vi "Event Handle Loop_Origin Zero.vi"(8 "error in (no error)":errorcluster, 11 "QTab Class in":refnum<class "QTab Class.lvclass">) -> (0 "error out":errorcluster, 3 "QTab Class out":refnum<class "QTab Class.lvclass">)   [LabVIEW 2020, in "QTab.lvlib" / "QTab Class.lvclass"]
uses:
  QTab Class.lvclass
  <vilib>/Utility/miscctls.llb/LVPointTypeDef.ctl
  QTab Class.lvclass/QTab Class.ctl
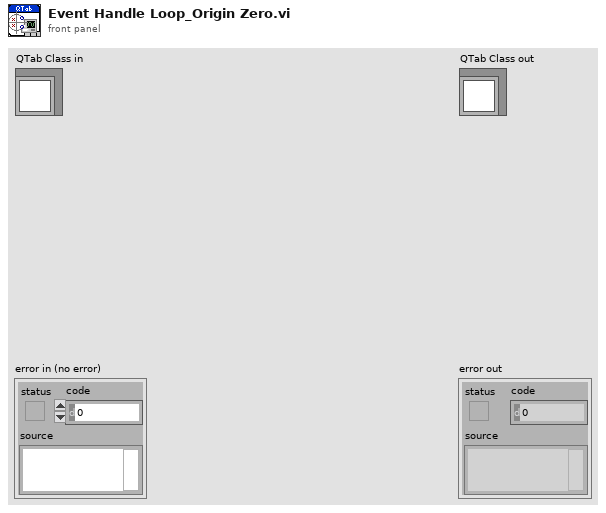
[diagram p1: front panel]
types:
  T1 = typedef "LVPointTypeDef.ctl" = cluster{"Horizontal":i16, "Vertical":i16}
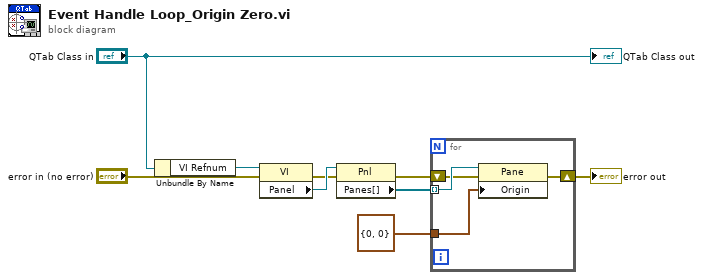
[diagram p0: block diagram]
diagram:
  n1 = Unbundle By Name("QTab Class in") -> ("VI Refnum"=w3:refnum<vi>)
  n2 = property class="VI"(reference=w3, error in="error in (no error)") -> (error out=w7:errorcluster, "Panel"=w9:refnum<vi>)  [unwired: 1 out]
  n3 = property class="Pnl"(reference=w9, error in=w7) -> (error out=w2:errorcluster, "Panes[]"=w8:refnum<vi>[])  [unwired: 1 out]
  n4 = for {
    tunnel: w8 -> [w13] mode=indexing
    shift-right: [w12] -> w1
    shift-left: w2 -> [w11]
    tunnel: T1 {"Horizontal"=0, "Vertical"=0} ("Origin") -> [w10]
    n5 = property class="Pane"(reference=w13, error in=w11, "Origin"=w10) -> (error out=w12:errorcluster)  [unwired: 1 out]
  }
  "error out" <- w1
  "QTab Class out" <- "QTab Class in"
